vi "GetMeasurements.vi"(8 "error in (no error)":errorcluster, 11 "ByteGSAPIBase in":refnum<class "ByteGSAPIBase.lvclass">) -> (0 "error out":errorcluster, 2 "Array":T1[](array[typedef]), 3 "ByteGSAPIBase out":refnum<class "ByteGSAPIBase.lvclass">)   [LabVIEW 2019, in "ByteGSWebAPI.lvlib" / "ByteGSAPIBase.lvclass"]
uses:
  ByteGSAPIBase.lvclass
  TypeDef/Measurement.ctl
  ByteGSAPIBase.lvclass/ByteGSAPIBase.ctl
  <vilib>/Bytelabs/ByteREST/ByteRESTClass/ByteRESTBase/RESTBase.lvclass
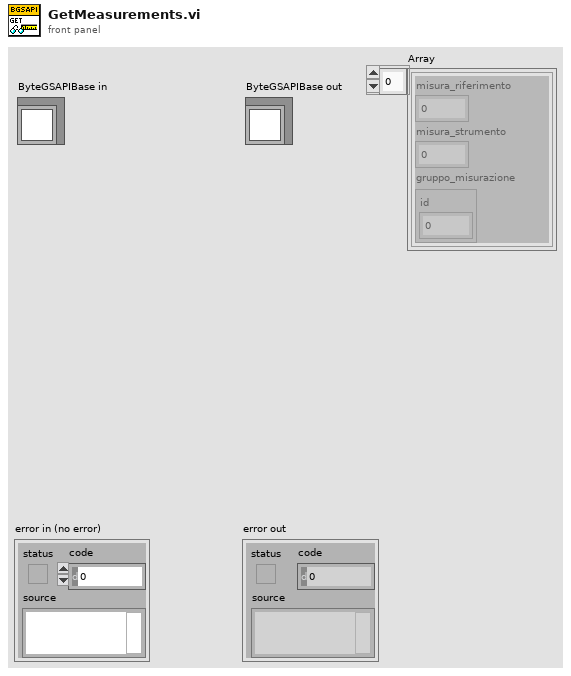
[diagram p1: front panel]
types:
  T1 = typedef "ByteGSWebAPI.lvlib/ByteGSAPIBase.lvclass/Measurement.ctl" = cluster{"misura_riferimento":sgl, "misura_strumento":sgl, "gruppo_misurazione":cluster{"id":u16}}
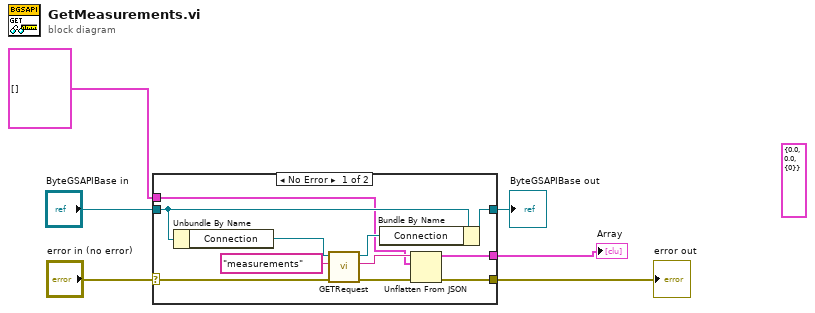
[diagram p0: block diagram]
diagram:
  (unwired) T1 {"misura_riferimento"=0.0, "misura_strumento"=0.0, "gruppo_misurazione"={"id"=0}} ("Valori")
  n1 = case shown="No Error" "error in (no error)" {
    selector: "error in (no error)" -> [w9 w20]
    tunnel: [w8 w20] -> w3
    tunnel: T1[] [] -> [w7 w19]
    tunnel: [w10 w19] -> w1
    tunnel: [w14 w18] -> w4
    tunnel: "ByteGSAPIBase in" -> [w17 w18]
    frame No Error {
      n2 = Unbundle By Name(w17) -> ("Connection"=w16:refnum<class "RESTBase.lvclass">)
      n3 = call-dynamic "GETRequest.vi"("error in (no error)"=w9, "Request"="measurements", "ByteRESTBase in"=w16) -> ("error out"=w15:errorcluster, "Body"=w11:string, "ByteRESTBase out"=w13:refnum<class "RESTBase.lvclass">)  [unwired: 5 in, 1 out]
      n4 = Bundle By Name(cluster=w17, "Connection"=w13) -> (w14:refnum<class "ByteGSAPIBase.lvclass">)
      n5 = Unflatten From JSON(JSON string=w11, type and defaults=w7, error in (no error)=w15) -> (value=w10:T1[], error out=w8:errorcluster)  [unwired: 4 in]
    }
    frame Error {
    }
  }
  "error out" <- w3
  "ByteGSAPIBase out" <- w4
  "Array" <- w1
